vi "Example_Counter_AO_2DAQ.vi"() -> ()   [LabVIEW 2025]
uses:
  <vilib>/DAQmx/write.llb/DAQmx Write (Analog Wfm 1Chan NSamp).vi
  <vilib>/Waveform/WDTOps.llb/WDT Number of Waveform Samples DBL.vi
  <vilib>/DAQmx/create/channels.llb/DAQmx Create Channel (CO-Pulse Generation-Time).vi
  <vilib>/DAQmx/configure/events/hardwareSignals.llb/DAQmx Export Signal (Most Signals).vi
  <vilib>/DAQmx/create/channels.llb/DAQmx Create Channel (AO-Voltage-Basic).vi
  <vilib>/DAQmx/configure/timing.llb/DAQmx Timing (Sample Clock).vi
  <vilib>/DAQmx/configure/trigger.llb/DAQmx Start Trigger (Digital Edge).vi
  <vilib>/DAQmx/miscellaneous.llb/DAQmx Fill In Error Info.vi
  <vilib>/measure/NI_MABase.lvlib
panel:
  out "error out":errorcluster
  out "Waveform Graph":waveform(dbl)(graph)
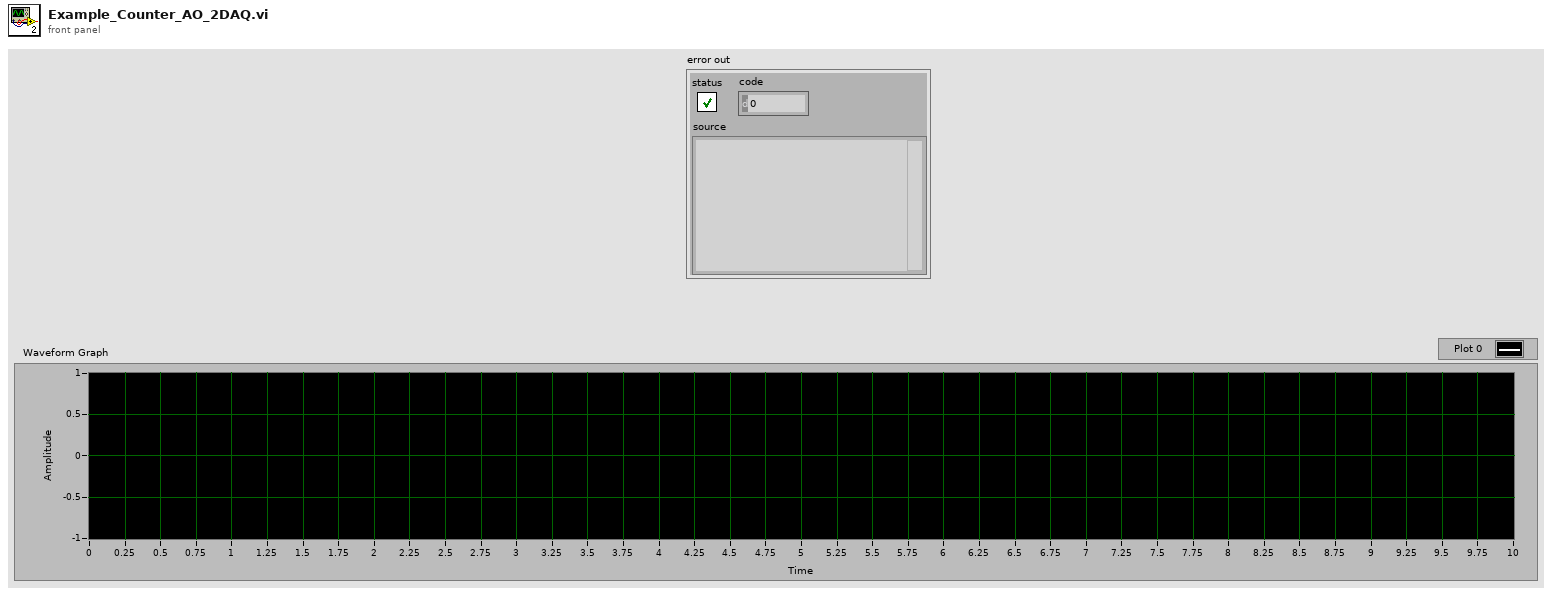
[diagram p1: front panel]
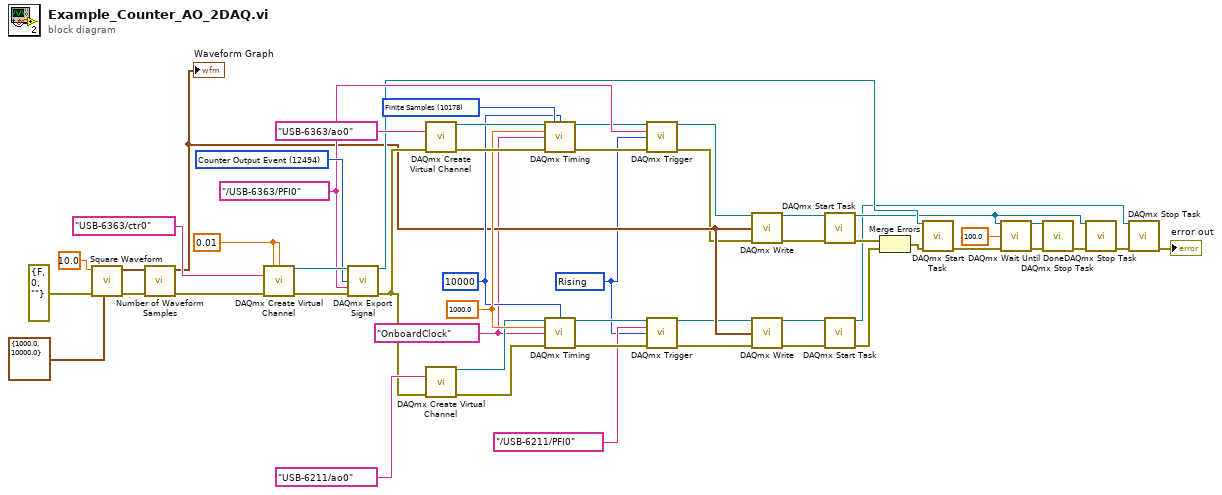
[diagram p0: block diagram]
diagram:
  w1 = 10280 items=["Rising"=10280, "Falling"=10171] ("edge")
  w21 = 10000 ("samples per channel")
  w45 = 10178 items=["Finite Samples"=10178, "Continuous Samples"=10123, "Hardware Timed Single Point"=12522] ("sample mode")
  w5 = tag "OnboardClock" ("source")
  w22 = 1000.0 ("rate")
  w44 = tag "/USB-6363/PFI0" ("output terminal")
  w48 = 12494 items=["AI Convert Clock"=12484, "10MHz Reference Clock"=12536, "20MHz Timebase Clock"=12486, "Sample Clock"=12487, "Advance Trigger"=12488, "Reference Trigger"=12490, "Start Trigger"=12491, "Advance Complete Event"=12492, "AI Hold Complete Event"=12493, "Counter Output Event"=12494, "Change Detection Event"=12511, "Watchdog Timer Expired Event"=12512] ("signal")
  w51 = 0.01 ("high time")
  n1 = call <vilib>:"Square Waveform.vi"("sampling info"=cluster{"Fs":dbl, "#s":dbl} {"Fs"=1000.0, "#s"=10000.0}, "error in (no error)"=errorcluster {"status"=FALSE, "code"=0, "source"=""}, "frequency"=10.0) -> ("error out"=w40:errorcluster, "signal out"=w41:waveform(dbl))  [unwired: 7 in]
  n2 = call-poly <vilib>:"Number of Waveform Samples.vi"("error in (no error)"=w40, "waveform in"=w41) -> ("error out"=w3:errorcluster, "waveform out"=w18:waveform(dbl))  [unwired: 7 in, 1 out]
  "Waveform Graph" <- w18
  n3 = call-poly <vilib>:"DAQmx Create Virtual Channel.vi"("high time"=w51, "low time"=w51, "counter"=tag "USB-6363/ctr0", "error in"=w3) -> ("task out"=w49:refnum<k21>, "error out"=w47:errorcluster)  [unwired: 10 in]
  n4 = call-poly <vilib>:"DAQmx Export Signal.vi"("task/channels in"=w49, "signal"=w48, "output terminal"=w44, "error in"=w47) -> ("task out"=w32:refnum<k21>, "error out"=w27:errorcluster)  [unwired: 10 in]
  n5 = call-poly <vilib>:"DAQmx Create Virtual Channel.vi"("physical channels"=tag "USB-6363/ao0", "error in"=w27) -> ("task out"=w26:refnum<k21>, "error out"=w28:errorcluster)  [unwired: 12 in]
  n6 = call-poly <vilib>:"DAQmx Create Virtual Channel.vi"("physical channels"=tag "USB-6211/ao0", "error in"=w27) -> ("task out"=w11:refnum<k21>, "error out"=w23:errorcluster)  [unwired: 12 in]
  n7 = call-poly <vilib>:"DAQmx Timing.vi"("task/channels in"=w26, "sample mode"=w45, "samples per channel"=w21, "rate"=w22, "source"=w5, "error in"=w28) -> ("task out"=w25:refnum<k21>, "error out"=w24:errorcluster)  [unwired: 8 in]
  n8 = call-poly <vilib>:"DAQmx Timing.vi"("task/channels in"=w11, "samples per channel"=w21, "rate"=w22, "source"=w5, "error in"=w23) -> ("task out"=w10:refnum<k21>, "error out"=w9:errorcluster)  [unwired: 9 in]
  n9 = call-poly <vilib>:"DAQmx Trigger.vi"("task/channels in"=w25, "source"=w44, "edge"=w1, "error in"=w24) -> ("task out"=w33:refnum<k21>, "error out"=w2:errorcluster)  [unwired: 10 in]
  n10 = call-poly <vilib>:"DAQmx Trigger.vi"("task/channels in"=w10, "source"=tag "/USB-6211/PFI0" ("output terminal"), "edge"=w1, "error in"=w9) -> ("task out"=w7:refnum<k21>, "error out"=w8:errorcluster)  [unwired: 10 in]
  n11 = call-poly <vilib>:"DAQmx Write.vi"("task/channels in"=w33, "data"=w18, "error in"=w2) -> ("task out"=w35:refnum<k21>, "error out"=w34:errorcluster)  [unwired: 10 in, 1 out]
  n12 = call-poly <vilib>:"DAQmx Write.vi"("task/channels in"=w7, "data"=w18, "error in"=w8) -> ("task out"=w19:refnum<k21>, "error out"=w20:errorcluster)  [unwired: 10 in, 1 out]
  n13 = call <vilib>:"DAQmx Start Task.vi"("task/channels in"=w35, "error in"=w34) -> ("task out"=w31:refnum<k21>, "error out"=w17:errorcluster)  [unwired: 12 in]
  n14 = call <vilib>:"DAQmx Start Task.vi"("task/channels in"=w19, "error in"=w20) -> ("task out"=w14:refnum<k21>, "error out"=w16:errorcluster)  [unwired: 12 in]
  n15 = Merge Errors(w17, w16) -> (w15:errorcluster)
  n16 = call <vilib>:"DAQmx Start Task.vi"("task/channels in"=w32, "error in"=w15) -> ("error out"=w37:errorcluster)  [unwired: 12 in, 1 out]
  n17 = call <vilib>:"DAQmx Wait Until Done.vi"("task/channels in"=w31, "timeout (sec)"=100.0, "error in"=w37) -> ("task out"=w39:refnum<k21>, "error out"=w38:errorcluster)  [unwired: 11 in]
  n18 = call <vilib>:"DAQmx Stop Task.vi"("task/channels in"=w39, "error in"=w38) -> ("error out"=w36:errorcluster)  [unwired: 12 in, 1 out]
  n19 = call <vilib>:"DAQmx Stop Task.vi"("task/channels in"=w31, "error in"=w36) -> ("error out"=w13:errorcluster)  [unwired: 12 in, 1 out]
  n20 = call <vilib>:"DAQmx Stop Task.vi"("task/channels in"=w14, "error in"=w13) -> ("error out"=→"error out":errorcluster)  [unwired: 12 in, 1 out]
